vi "Raster.vi"(4 "Draw Lines":bool, 5 "Draw Triangles":bool, 6 "Line Colour":u32(colorbox)=4375295, 7 "Textured":bool, 10 "Triangles Sorted":T1[](array[typedef]) {"Vertex 3"."UV"."v" min=0 max=1 step=0.1; "Vertex 3"."UV"."u" min=0 max=1 step=0.1; "Vertex 2"."UV"."v" min=0 max=1 step=0.1; "Vertex 2"."UV"."u" min=0 max=1 step=0.1; "Vertex 1"."UV"."v" min=0 max=1 step=0.1; "Vertex 1"."UV"."u" min=0 max=1 step=0.1}, 11 "Pixel Data in":u32[][](array[numeric])) -> (3 "Pixel Data out":u32[][](array[numeric]))   [LabVIEW 2020, in "3D (FPGA).lvlib"]
uses:
  3D (FPGA).lvlib
  Raster/Raster (FPGA).lvlib
  Raster/UV.ctl
  Raster/Rectangle Dimensions.ctl
  Raster/Texture.ctl
  Vector 3D.ctl
  Vertex.ctl
  Triangle.ctl
  Material.ctl
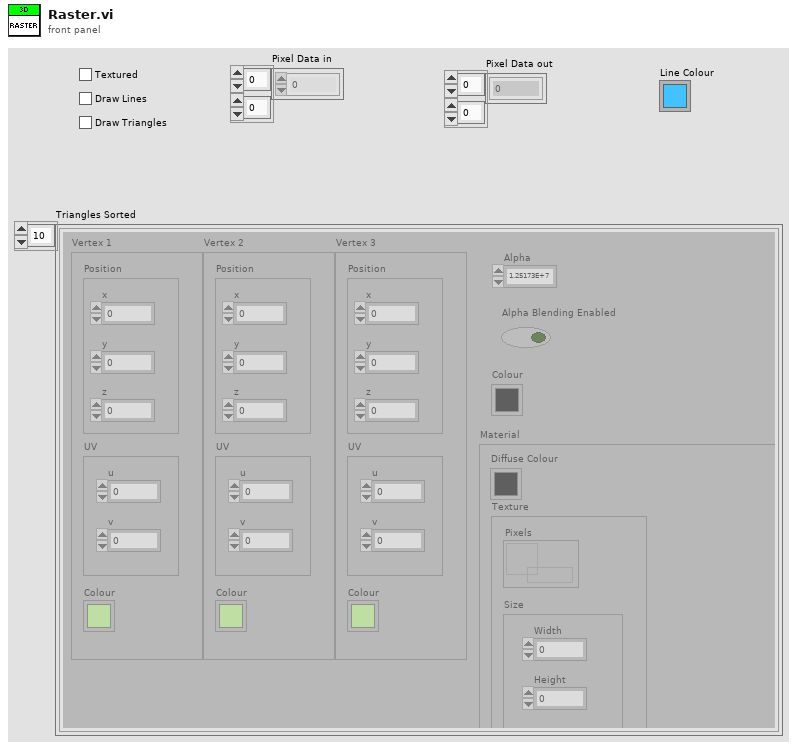
[diagram p1: front panel]
types:
  T1 = typedef "3D (FPGA).lvlib/Triangle.ctl" = cluster{"Vertex 1":T2, "Vertex 2":T2, "Vertex 3":T2, "Alpha":dbl, "Alpha Blending Enabled":bool, "Colour":u32, "Material":T5}
  T2 = typedef "3D (FPGA).lvlib/Vertex.ctl" = cluster{"Position":T3, "UV":T4, "Colour":u32}
  T3 = typedef "3D (FPGA).lvlib/Vector 3D.ctl" = cluster{"x":sgl, "y":sgl, "z":sgl}
  T4 = typedef "Raster (FPGA).lvlib/UV.ctl" = cluster{"u":sgl, "v":sgl}
  T5 = typedef "3D (FPGA).lvlib/Material.ctl" = cluster{"Diffuse Colour":u32, "Texture":T6}
  T6 = typedef "Raster (FPGA).lvlib/Texture.ctl" = cluster{"Pixels":refnum<data-value>, "Size":T7}
  T7 = typedef "Raster (FPGA).lvlib/Rectangle Dimensions.ctl" = cluster{"Width":u32, "Height":u32}
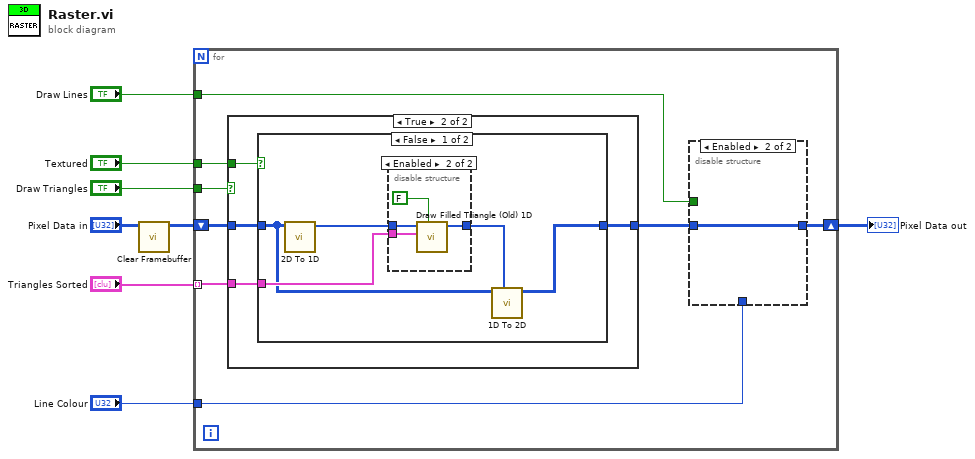
[diagram p0: block diagram]
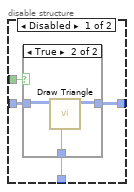
[diagram p2: hidden frame]
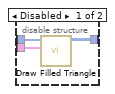
[diagram p5: hidden frame]
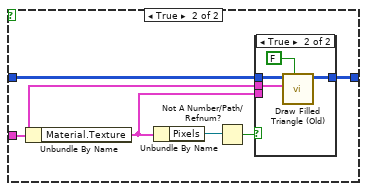
[diagram p6: hidden frame]
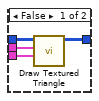
[diagram p7: hidden frame]
diagram:
  n1 = call "Clear Framebuffer.vi"("Pixel Data in"="Pixel Data in") -> ("Pixel Data out"=w4:u32[][])  [unwired: 10 in]
  n2 = for {
    tunnel: "Line Colour" -> [w16]
    tunnel: "Triangles Sorted" -> [w10] mode=indexing
    tunnel: "Draw Lines" -> [w15]
    tunnel: "Draw Triangles" -> [w12]
    shift-right: [w11] -> w2
    shift-left: w4 -> [w14]
    tunnel: "Textured" -> [w9]
    n3 = case shown="True" w12 {
      tunnel: w14 -> [w26 w30]
      tunnel: [w26 w29] -> w13
      tunnel: w10 -> [_ w28]
      tunnel: w9 -> [_ w27]
      frame False {
      }
      frame True {
        n4 = case shown="False" w27 {
          tunnel: w30 -> [w33 w48]
          tunnel: [w31 w47] -> w29
          tunnel: w28 -> [w35 w46]
          frame False {
            n5 = call "2D To 1D.vi"("Pixel Data in"=w33) -> ("1D Pixel Data out"=w34:u32[])  [unwired: 10 in]
            n6 = disable-structure shown="Enabled" {
              disable-tunnel: w34 -> [w38 w42]
              disable-tunnel: [w37 w41] -> w32
              disable-tunnel: w35 -> [w36 w40]
              frame Disabled {
                n7 = call "Draw Filled Triangle.vi"("Triangle"=w36, "Pixel Data in"=w38) -> ("Pixel Data out"=w37:u32[][])  [unwired: 9 in]
              }
              frame Enabled {
                n8 = call "Draw Filled Triangle (Old) 1D.vi"("Enable Alpha Blending (F)"=FALSE, "Triangle"=w40, "Pixel Data in"=w42) -> ("Pixel Data out"=w41:u32[])  [unwired: 8 in]
              }
            }
            n9 = call "1D To 2D.vi"("1D Pixel Data in"=w32, "2D Pixel Data in"=w33) -> ("2D Pixel Data out"=w31:u32[][])  [unwired: 9 in]
          }
          frame True {
            n10 = Unbundle By Name(w46) -> ("Material.Texture"=w45:T6)
            n11 = Unbundle By Name(w45) -> ("Pixels"=w44:refnum<data-value>)
            n12 = Not A Number/Path/Refnum?(number/path/refnum=w44) -> (NaN/Path/Refnum?=w43:bool)
            n13 = case shown="True" w43 {
              tunnel: w48 -> [w52 w55]
              tunnel: [w51 w54] -> w47
              tunnel: w46 -> [w50 w53]
              tunnel: w45 -> [w49 _]
              frame False {
                n14 = call "Draw Textured Triangle.vi"("Texture"=w49, "Triangle"=w50, "Pixel Data in"=w52) -> ("Pixel Data out"=w51:u32[][])  [unwired: 8 in]
              }
              frame True {
                n15 = call "Draw Filled Triangle (Old).vi"("Enable Alpha Blending (F)"=FALSE, "Triangle"=w53, "Pixel Data in"=w55) -> ("Pixel Data out"=w54:u32[][])  [unwired: 8 in]
              }
            }
          }
        }
      }
    }
    n16 = disable-structure shown="Enabled" {
      disable-tunnel: w16 -> [w20 _]
      disable-tunnel: w15 -> [w19 _]
      disable-tunnel: w13 -> [w18 w25]
      disable-tunnel: [w17 w25] -> w11
      frame Disabled {
        n17 = case shown="True" w19 {
          tunnel: w18 -> [w21 w23]
          tunnel: w20 -> [_ w24]
          tunnel: [w21 w22] -> w17
          frame False {
          }
          frame True {
            n18 = call "Draw Triangle.vi"("Line Colour"=w24, "Pixel Data in"=w23) -> ("Pixel Data out"=w22:u32[][])  [unwired: 9 in]
          }
        }
      }
      frame Enabled {
      }
    }
  }
  "Pixel Data out" <- w2
